vi "groß oder klein.vi"(8 "error in (no error)":errorcluster caption="Fehler (Eingang, kein Fehler)", 11 "Device ID":T1(ring)) -> (0 "error out":errorcluster caption="Fehler (Ausgang)", 2 "Groß?":bool, 3 "Device ID Out":T1(ring))   [LabVIEW 2010]
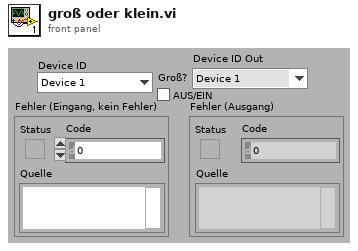
[diagram p1: front panel]
types:
  T1 = enum16{"Device 1", "Device 2", "Device 3", "Device 4", "Device 5", "Device 6", "Device 7", "Device 8"}
  T2 = enum8{"Power 1", "Power 2", "Power 3", "Power 4", "Power 5", "Power 6", "Power 7", "Power 8"}
  T3 = enum8{"Output 1 (O1)", "Output 2 (O2)", "Output 3 (O3)", "Output 4 (O4)", "Output 5 (O5)", "Output 6 (O6)", "Output 7 (O7)", "Output 8 (O8)"}
  T4 = enum8{"Robo Interface", "Extension 1", "Extension 2", "Extension 3"}
  T5 = enum8{"Input 1 (I1)", "Input 2 (I2)", "Input 3 (I3)", "Input 4 (I4)", "Input 5 (I5)", "Input 6 (I6)", "Input 7 (I7)", "Input 8 (I8)"}
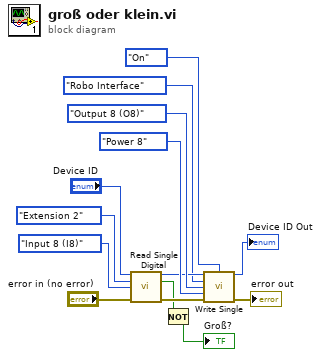
[diagram p0: block diagram]
diagram:
  n1 = call "Read Single Digital.vi"("Device ID"="Device ID", "Module"=T4."Extension 2", "Digital_Input"=T5."Input 8 (I8)", "error in"="error in (no error)") -> ("Device ID Out"=w8:T1, "Value"=w6:bool, "error out"=w11:errorcluster)  [unwired: 9 out]
  n2 = Not(x=w6) -> (.not. x?=→"Groß?":bool)
  n3 = call "Write Single.vi"("Device ID"=w8, "Output_Action"=enum8{"Off", "On"}."On", "Module"=T4."Robo Interface", "Single_Output"=T3."Output 8 (O8)", "Output_PWM"=T2."Power 8", "error in"=w11) -> ("Device ID Out"=→"Device ID Out":T1, "error out"=→"error out":errorcluster)  [unwired: 8 out]
